vi "WriteCase.vi"(7 "Iteration 1st loop":i16, 8 "error in (no error)":errorcluster, 9 "Iteration 2nd loop":i16, 10 "image data":T1, 11 "Current path":path) -> (0 "error out":errorcluster)   [LabVIEW 2020]
uses:
  <vilib>/picture/picture.llb/imagedata.ctl
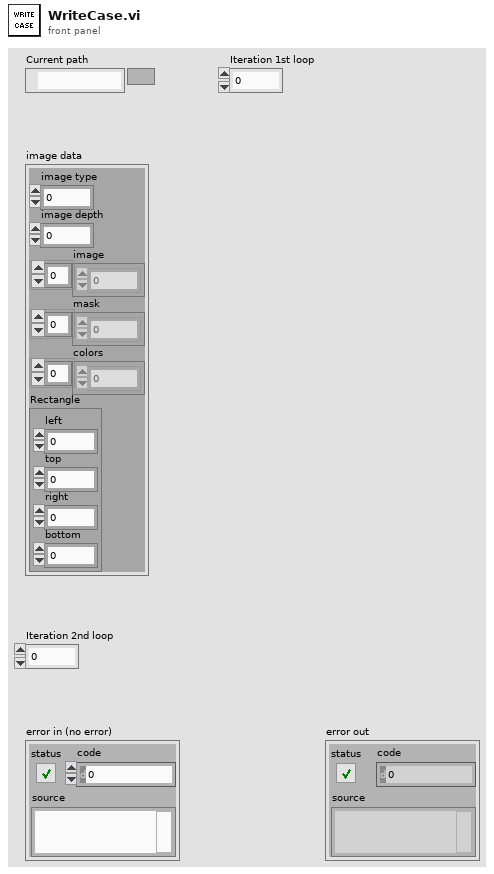
[diagram p1: front panel]
types:
  T1 = typedef "imagedata.ctl" = cluster{"image type":i32, "image depth":i32, "image":u8[], "mask":u8[], "colors":u32[], "Rectangle":cluster{"left":i16, "top":i16, "right":i16, "bottom":i16}}
  T2 = enum16{"big-endian, network order", "native, host order", "little-endian"}
  T3 = cluster{"left":i16, "top":i16, "right":i16, "bottom":u16}
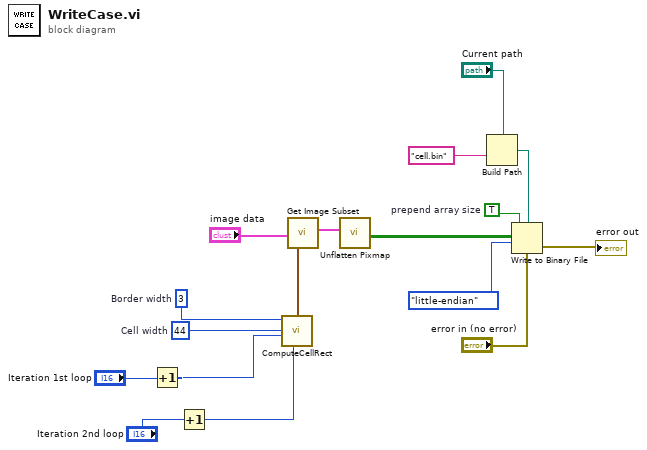
[diagram p0: block diagram]
diagram:
  w15 = 44  # Cell width
  w14 = 3  # Border width
  w11 = TRUE  # prepend array size
  n1 = Increment(x="Iteration 1st loop") -> (x+1=w1:i16)
  n2 = Increment(x="Iteration 2nd loop") -> (x+1=w3:i16)
  n3 = call "ComputeCellRect.vi"("Column"=w3, "Line"=w1, "Cell width"=w15, "Border width"=w14) -> ("Cell rect"=w16:T3)  [unwired: 7 in]
  n4 = call <vilib>:"Get Image Subset.vi"("subset rect"=w16, "image data"="image data") -> ("image subset"=w10:T1)  [unwired: 4 in, 1 out]
  n5 = call <vilib>:"Unflatten Pixmap.vi"("image data"=w10) -> ("1-bit pixmap"=w17:bool[][])  [unwired: 4 in, 6 out]
  n6 = Build Path(base path="Current path", name or relative path="cell.bin") -> (appended path=w6:path)
  n7 = Write to Binary File(file (use dialog)=w6, data=w17, error in="error in (no error)", 5:w11, 9:T2."little-endian" ("byte order")) -> (error out=→"error out":errorcluster)  [unwired: 1 in, 2 out]
